vi "Example_1.vi"() -> ()   [LabVIEW 2020, in "PixPack.lvlib"]
uses:
  PixPack.lvlib
  ce672bd1-fffe-424f-a641-cc0b68ed6e9e.vi
  <vilib>/Utility/error.llb/Clear Errors.vi
  private/MGI U8 Data to Hex Str.vi
  private/MGI Hex Str to U8 Data.vi
  <vilib>/Utility/error.llb/Error Cluster From Error Code.vi
  <vilib>/Utility/libraryn.llb/Get File Extension.vi
  private/PP.Encode.Decode.RC4.vi
  <vilib>/Utility/libraryn.llb/Generate Temporary File Path.vi
  private/PP.Create.PNG.By.ByteArray.vi
  <vilib>/picture/png.llb/Read PNG File.vi
panel:
  out "2D Picture":picture
  out "error out":errorcluster
  out "XML Out (if XML Flattened)":string
  out "Type of Encode":T1(ring)
  out "Value":T2(array[cluster])
  in  "error in":errorcluster
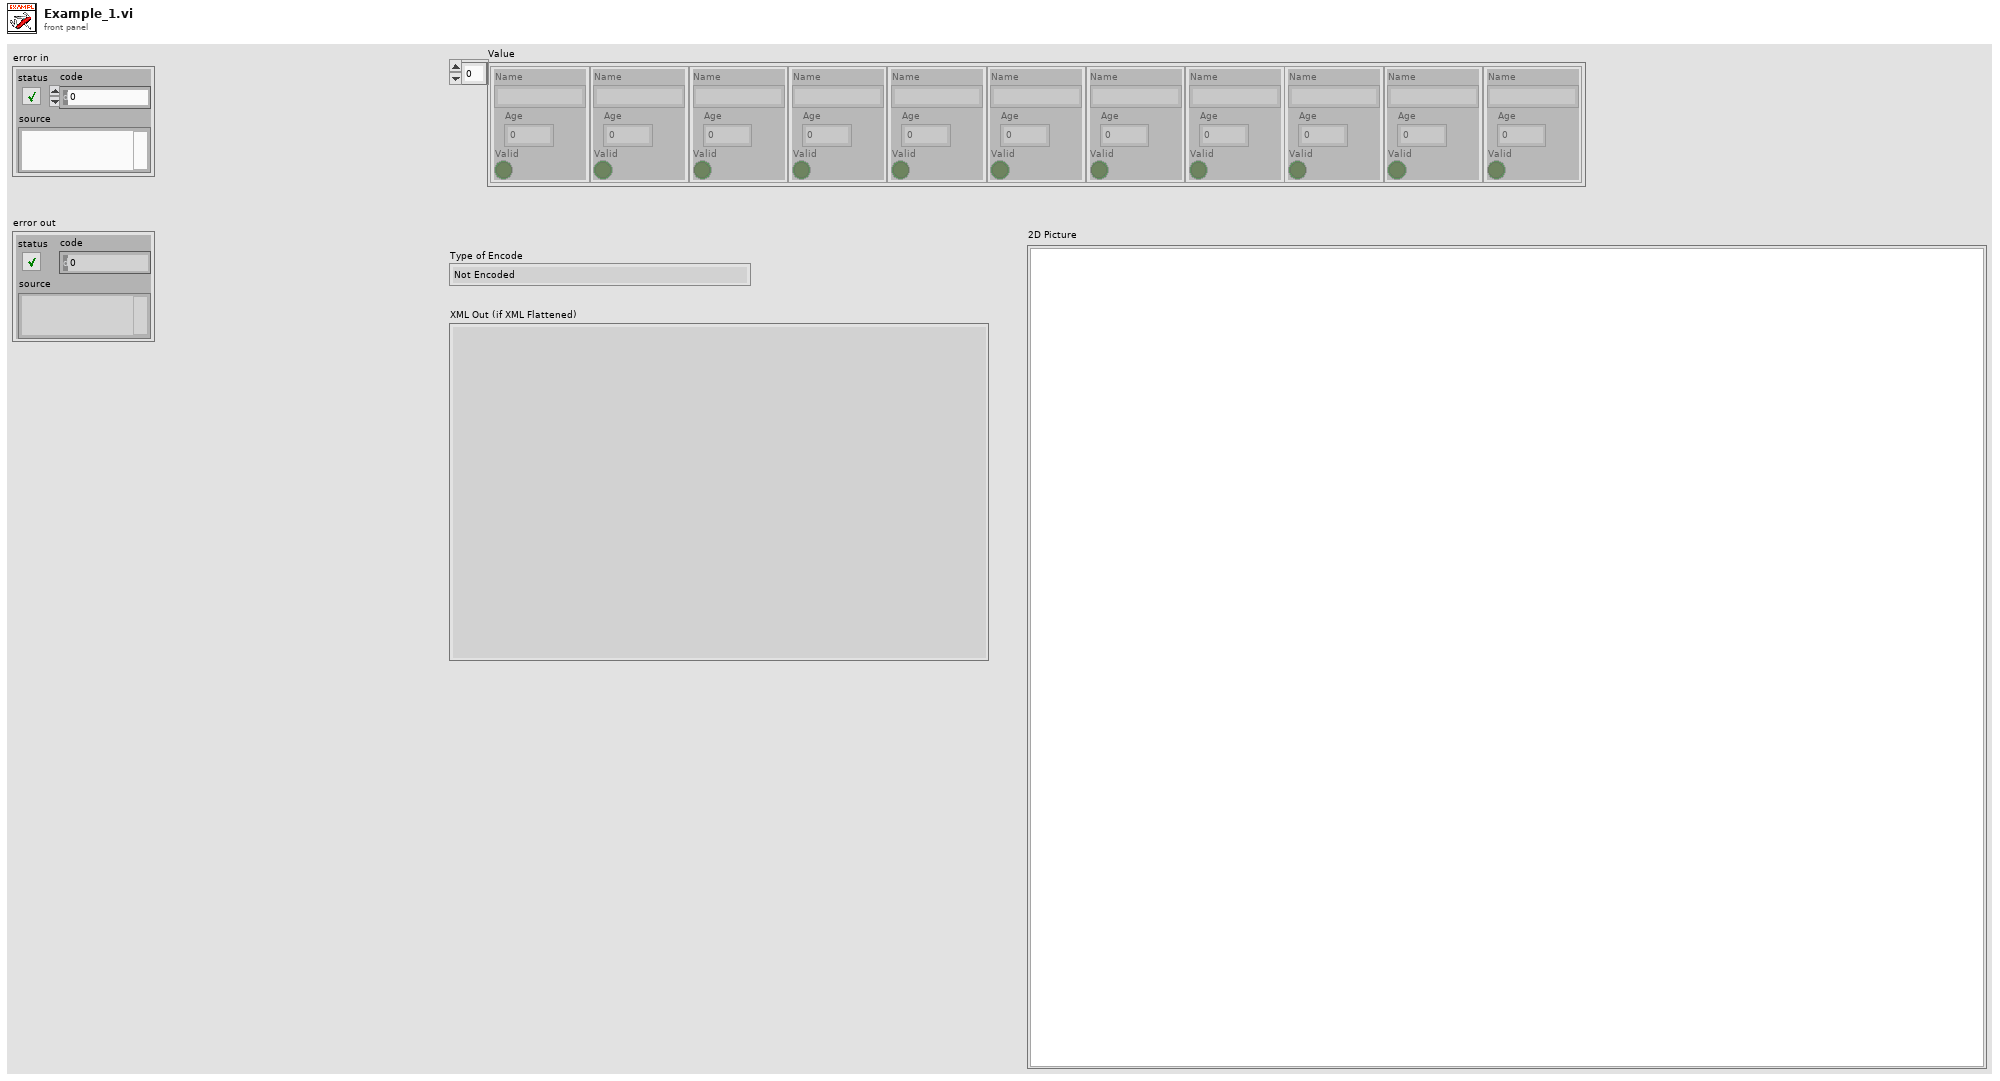
[diagram p1: front panel]
types:
  T1 = enum16{"Not Encoded", "Normal Flatten", "XML Flatten"}
  T2 = cluster{"Name":string, "Age":i32, "Valid":bool}[]
  T3 = typedef "imagedata.ctl" = cluster{"image type":i32, "image depth":i32, "image":u8[], "mask":u8[], "colors":u32[], "Rectangle":cluster{"left":i16, "top":i16, "right":i16, "bottom":i16}}
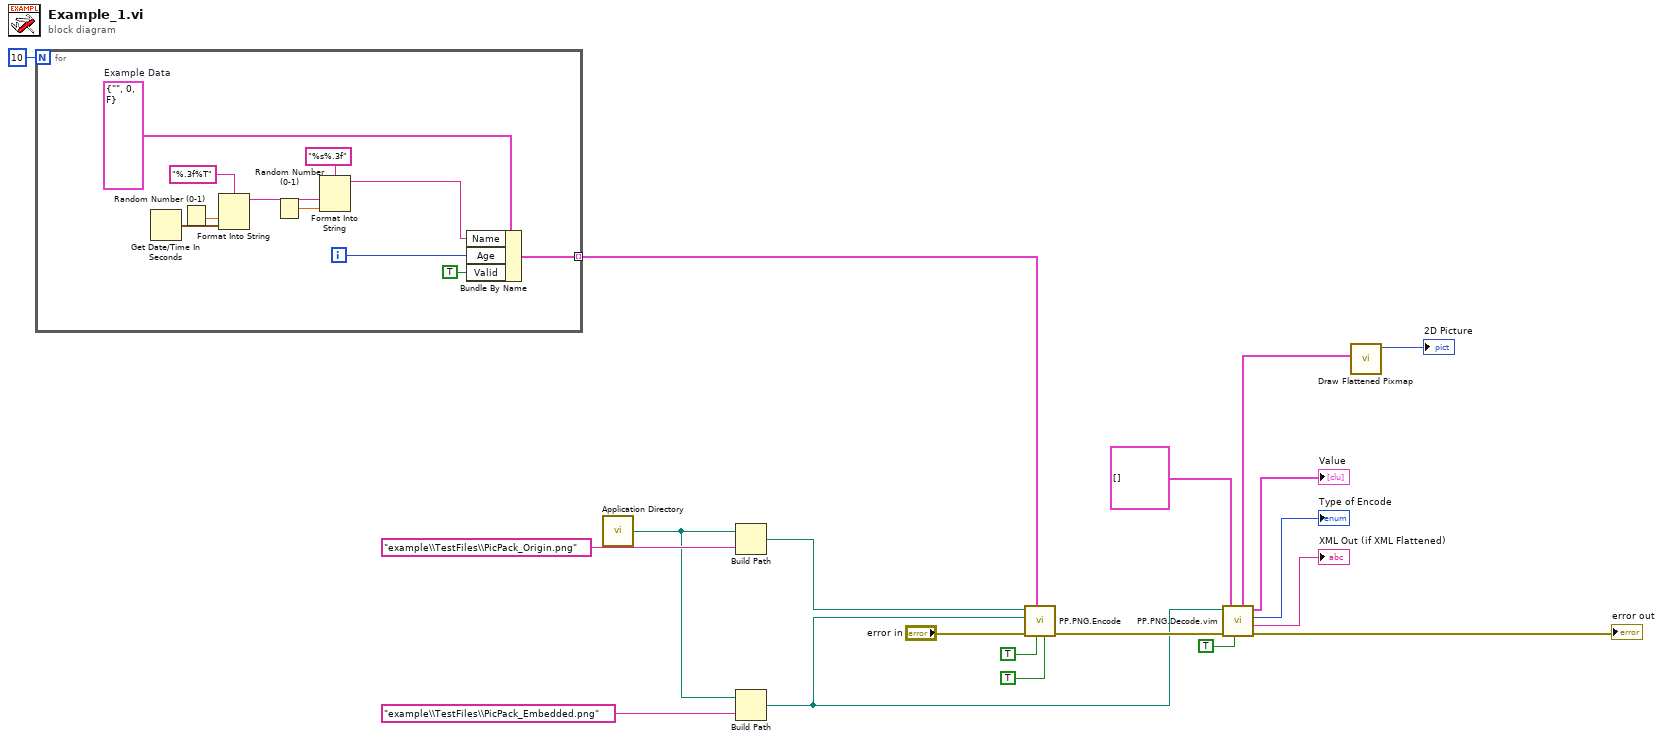
[diagram p0: block diagram]
diagram:
  n1 = for {
    N: 10 -> [_]
    tunnel: [w20] -> w1 mode=indexing
    i -> [w22]
    w24 = cluster{"Name":string, "Age":i32, "Valid":bool} {"Name"="", "Age"=0, "Valid"=FALSE}  # Example Data
    n2 = Get Date/Time In Seconds() -> (seconds since 1Jan1904=w28:timestamp)
    n3 = Random Number (0-1)() -> (number: 0 to 1=w29:dbl)
    n4 = Format Into String(format string="%.3f%T", w29, w28) -> (resulting string=w30:string)  [unwired: 2 in, 1 out]
    n5 = Random Number (0-1)() -> (number: 0 to 1=w25:dbl)
    n6 = Format Into String(format string="%s%.3f", w30, w25) -> (resulting string=w23:string)  [unwired: 2 in, 1 out]
    n7 = Bundle By Name(cluster=w24, "Name"=w23, "Age"=w22, "Valid"=TRUE) -> (w20:cluster{"Name":string, "Age":i32, "Valid":bool})
  }
  n8 = call <vilib>:"Application Directory.vi"() -> ("Application Directory"=w15:path)
  n9 = Build Path(base path=w15, name or relative path="example\\TestFiles\\PicPack_Origin.png") -> (appended path=w16:path)
  n10 = Build Path(base path=w15, name or relative path="example\\TestFiles\\PicPack_Embedded.png") -> (appended path=w13:path)
  n11 = call "PP.PNG.Encode.vi"("Data Owerwrite (T)"=TRUE, "XML Encode (F)"=TRUE, "Data"=w1, "error in"="error in", "Destination PNG (default: empty)"=w13, "PNG In"=w16) -> ("error out"=w17:errorcluster)  [unwired: 5 in]
  n12 = call "PP.PNG.Decode.vim"("Get Image Data (F)"=TRUE, "Data Type (Default)"=T2 [] ("appended array"), "error in"=w17, "PNG In"=w13) -> ("error out"=→"error out":errorcluster, "XML Out (if XML Flattened)"=→"XML Out (if XML Flattened)":string, "Type of Encode"=→"Type of Encode":T1, "Value"=→"Value":T2, "Image Data"=w6:T3)  [unwired: 3 in]
  n13 = call <vilib>:"Draw Flattened Pixmap.vi"("image data"=w6) -> ("new picture"=→"2D Picture":picture)  [unwired: 8 in]
